vi "VIew VI's Color Palette.vi"() -> ()   [LabVIEW 2021]
doc: "Launch the View-User Colors Palette VI through the tools menu if the theme data is saved as part of the tag data for the VI.\n\n<b>Code Developed By:</b> +\nDaniel Coons +\nTechnology Service Corporation +\nwww.tsc.com/atcs"
uses:
  Material SubVIs/Material SubVIs.lvlib
  Material Theme/Material Theme.lvclass
  Material-Scheme/Material-Scheme.lvclass
panel:
  in  "color":bool
  # "Load the Palette..."
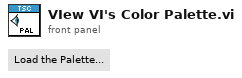
[diagram p1: front panel]
types:
  T1 = enum32{"Invalid", "Standard", "Closed", "Hidden", "Minimized", "Maximized"}
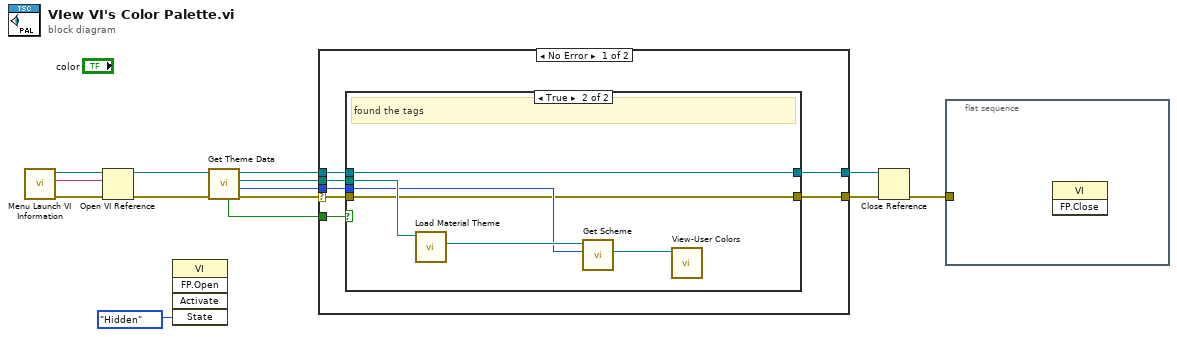
[diagram p0: block diagram]
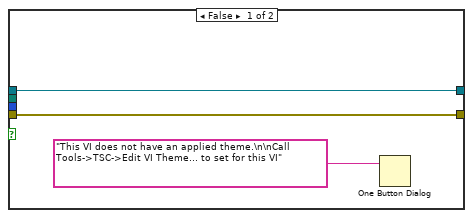
[diagram p2: hidden frame]
diagram:
  n1 = call <vilib>:"Menu Launch VI Information.vi"() -> ("error out"=w12:errorcluster, "Menu Launch:VI"=w13:string, "Menu Launch:App"=w14:refnum<vi>)  [unwired: 9 in]
  n2 = Open VI Reference(application reference (local)=w14, vi path=w13, error in (no error)=w12) -> (vi reference=w11:refnum<vi>, error out=w10:errorcluster)  [unwired: 3 in]
  n3 = invoke class="VI" method="FP.Open"("State"=T1."Hidden") -> ()  [unwired: 4 in, 5 out]
  n4 = call "Get Theme Data.vi"("error in"=w10, "VI Refnum"=w11) -> ("error out"=w9:errorcluster, "Theme"=w3:u16, "Theme Path"=w4:path, "VI Refnum out"=w8:refnum<vi>, "Found?"=w5:bool)  [unwired: 5 in]
  n5 = case shown="No Error" w9 {
    selector: w9 -> [w21 w32]
    tunnel: w8 -> [w18 w31]
    tunnel: [w15 w32] -> w7
    tunnel: [w16 w31] -> w6
    tunnel: w5 -> [w20 _]
    tunnel: w4 -> [w19 _]
    tunnel: w3 -> [w17 _]
    frame No Error {
      n6 = case shown="True" w20 {
        tunnel: w21 -> [w23 w25]
        tunnel: w19 -> [_ w30]
        tunnel: w18 -> [w24 w29]
        tunnel: w17 -> [_ w27]
        tunnel: [w24 w29] -> w16
        tunnel: [w23 w25] -> w15
        frame False {
          n7 = One Button Dialog(message="This VI does not have an applied theme.\n\nCall Tools->TSC->Edit VI Theme... to set for this VI") -> ()  [unwired: 1 in, 1 out]
        }
        frame True {
          # "found the tags"
          n8 = call "Load Material Theme.vi"("file path"=w30) -> ("Theme"=w28:refnum<class "Material Theme.lvclass">)  [unwired: 8 in, 2 out]
          n9 = call "Get Scheme.vi"("Theme"=w27, "Material Theme in"=w28) -> ("Material-Scheme"=w26:refnum<class "Material-Scheme.lvclass">)  [unwired: 7 in, 2 out]
          n10 = call "View-User Colors.vi"("Material-Scheme.lvclass"=w26) -> ()  [unwired: 11 in]
        }
      }
    }
    frame Error {
    }
  }
  n11 = Close Reference(reference=w6, error in (no error)=w7) -> (error out=w2:errorcluster)
  n12 = flat-sequence {
    tunnel: w2 -> [_]
    frame #0 {
      n13 = invoke class="VI" method="FP.Close"() -> ()  [unwired: 3 in, 3 out]
    }
  }
